vi "Close stage.vi"(8 "error in":errorcluster) -> (0 "error out":errorcluster)   [LabVIEW 2017]
uses:
  MCM3000/LabVIEW/inc/MCM3000.lvlib
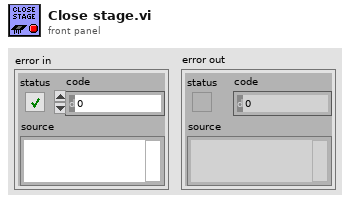
[diagram p1: front panel]
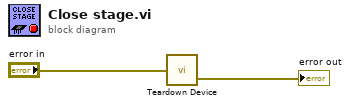
[diagram p0: block diagram]
diagram:
  n1 = call "Teardown Device.vi"("error in (no error)"="error in") -> ("error out"=→"error out":errorcluster)  [unwired: 1 out]
